vi "Filter.vi"(11 "dataflow in":T1) -> (3 "dataflow out":T1)   [LabVIEW 2018, in "GLog.lvlib" / "Logger.lvclass"]
uses:
  Logger.lvclass
  213feef3-c00a-4a99-bc2f-537bf3ca403c.vi
  Utilities/Panic.vi
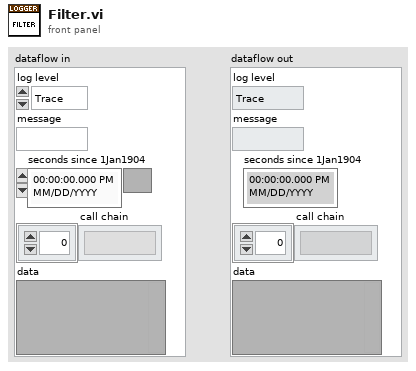
[diagram p1: front panel]
types:
  T1 = cluster{"log level":enum16{"Trace", "Debug", "Info", "Warning", "Error", "Critical"}, "message":string, "seconds since 1Jan1904":timestamp, "call chain":string[], "data":variant}
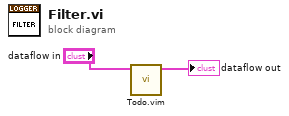
[diagram p0: block diagram]
diagram:
  n1 = call "Todo.vim"("dataflow in"="dataflow in") -> ("dataflow out"=→"dataflow out":T1)  [unwired: 10 in]
